vi "TotalScanTime2RB (SubVI).vi"(11 "NTick":i32) -> (3 "T_sum":dbl format="%0.2f")   [LabVIEW 2017]
uses:
  Global_SNK3_HF.vi
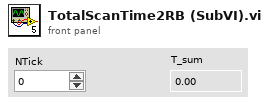
[diagram p1: front panel]
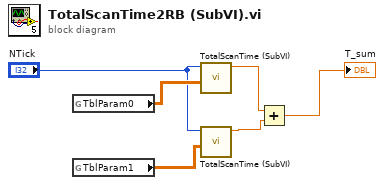
[diagram p0: block diagram]
diagram:
  n1 = global read "Global_SNK3_HF.vi" "TblParam0"() -> (w6:sgl[][])
  n2 = global read "Global_SNK3_HF.vi" "TblParam1"() -> (w5:sgl[][])
  n3 = call "TotalScanTime (SubVI).vi"("TblParam"=w6, "NTick"="NTick") -> ("sum"=w3:dbl)  [unwired: 9 in]
  n4 = call "TotalScanTime (SubVI).vi"("TblParam"=w5, "NTick"="NTick") -> ("sum"=w2:dbl)  [unwired: 9 in]
  n5 = Add(x=w3, y=w2) -> (x+y=→"T_sum":dbl)
